vi "Send Command.vi"(8 "error in (no error)":errorcluster, 10 "Command":string, 11 "RSeries_CAM in":refnum<class "RSeries_CAM.lvclass">) -> (0 "error out":errorcluster, 1 "Response":string, 2 "Success?":bool, 3 "RSeries_CAM out":refnum<class "RSeries_CAM.lvclass">)   [LabVIEW 2024, in "RSeries_CAM.lvlib" / "RSeries_CAM.lvclass"]
uses:
  RSeries_CAM.lvclass
  RSeries_CAM.lvclass/RSeries_CAM.ctl
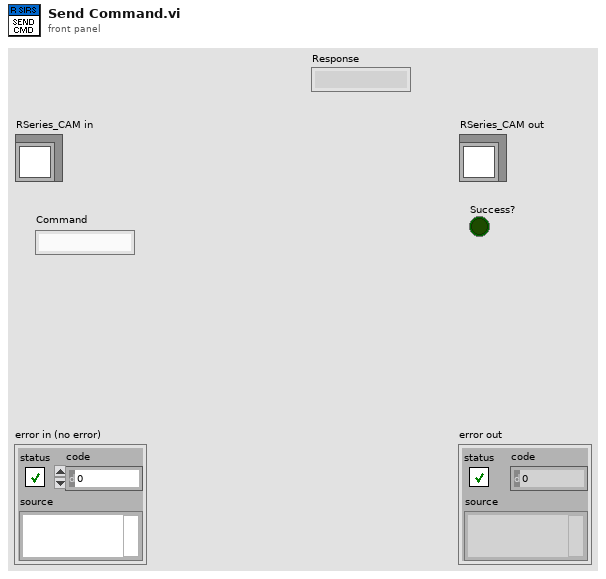
[diagram p1: front panel]
types:
  T1 = enum16{"Standard", "Buffered", "CRLF", "Immediate"}
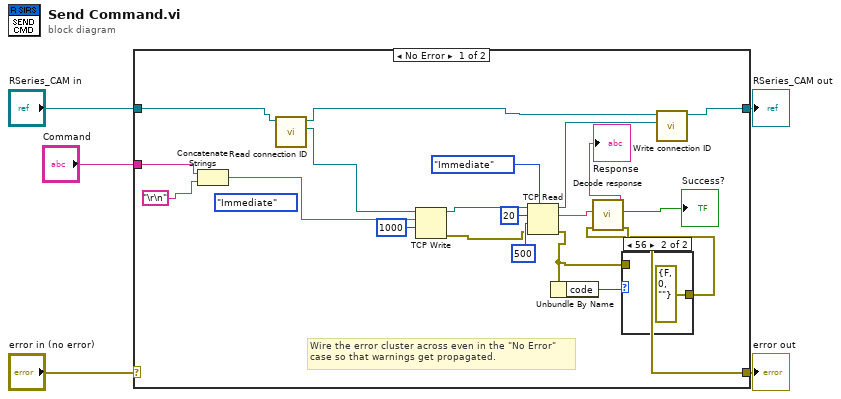
[diagram p0: block diagram]
diagram:
  n1 = case shown="No Error" "error in (no error)" {
    selector: "error in (no error)" -> [_ w30]
    tunnel: [w15 w30] -> w4
    tunnel: [w21 w29] -> w2
    tunnel: "RSeries_CAM in" -> [w26 w29]
    tunnel: "Command" -> [w25 _]
    frame No Error {
      (unwired) T1."Immediate" ("mode (standard)")
      # "Wire the error cluster across even in the \"No Error\"\ncase so that warnings get propagated."
      n2 = Concatenate Strings(w25, "\r\n") -> (w24:string)
      n3 = call "Read connection ID.vi"("RSeries_CAM in"=w26) -> ("connection ID"=w6:refnum<k5>, "RSeries_CAM out"=w22:refnum<class "RSeries_CAM.lvclass">)  [unwired: 8 in, 1 out]
      n4 = TCP Write(connection ID=w6, data in=w24, 9:1000 ("timeout ms (25000)")) -> (connection ID out=w20:refnum<k5>, error out=w17:errorcluster)  [unwired: 1 in, 1 out]
      n5 = TCP Read(connection ID=w20, bytes to read=20, error in (no error)=w17, 7:T1."Immediate" ("mode (standard)"), 9:500 ("timeout ms (25000)")) -> (connection ID out=w16:refnum<k5>, data out=w10:string, error out=w7:errorcluster)
      n6 = Unbundle By Name(w7) -> ("code"=w9:i32)
      n7 = case shown="56" w9 {
        tunnel: [w27 errorcluster {"status"=FALSE, "code"=0, "source"=""} ("error out")] -> w8
        tunnel: w7 -> [w27 _]
        frame 0, Default {
        }
        frame 56 {
        }
      }
      n8 = call "Decode response.vi"("error in (no error)"=w8, "Recieved"=w10) -> ("error out"=w15:errorcluster, "Command Accepted"=→"Success?":bool, "Remainning response"=→"Response":string)  [unwired: 7 in]
      n9 = call "Write connection ID.vi"("connection ID"=w16, "RSeries_CAM in"=w22) -> ("RSeries_CAM out"=w21:refnum<class "RSeries_CAM.lvclass">)  [unwired: 8 in, 1 out]
    }
    frame Error {
    }
  }
  "error out" <- w4
  "RSeries_CAM out" <- w2
